vi "Data_Acquisition(I&O).vi"() -> ()   [LabVIEW 2020]
uses:
  <vilib>/Platform/TimedLoop/XDataNode/timing_clust.ctl
  <vilib>/Platform/TimedLoop/XDataNode/nitl_modes.ctl
  <vilib>/Platform/TimedLoop/XDataNode/wakeup.ctl
  <vilib>/FPGAPlugInAG/cRIO-9047/niLvFpga_Open_cRIO-9047.vi
  <vilib>/rvi/interface/common/dynamic/niFpgaDynamicAddResources.vi
  <vilib>/FPGAPlugInAG/Dynamic/niLvFpga_Download_Dynamic.vi
  <vilib>/FPGAPlugInAG/Dynamic/niLvFpga_Reset_Dynamic.vi
  <vilib>/FPGAPlugInAG/Dynamic/niLvFpga_Run_Dynamic.vi
  <vilib>/Utility/error.llb/Error Cluster From Error Code.vi
  <vilib>/rvi/errors/niLvFpgaAdjustHostInterfaceError.vi
  <vilib>/FPGAPlugInAG/Dynamic/niLvFpga_Close_Dynamic.vi
  <vilib>/Platform/TimedLoop/XDataNode/XDataNode.xnode
  <vilib>/rvi/interface/nirviOpenFPGA/nirviOpenFPGA.xnode
  FPGA_Link.vi
  <vilib>/rvi/interface/nirviMethod/nirviMethod.xnode
  <vilib>/rvi/interface/nirviReadWriteControl/nirviReadWriteControl.xnode
  <vilib>/rvi/interface/nirviCloseFPGA/nirviCloseFPGA.xnode
  <vilib>/Platform/TimedLoop/XDataNode/XDNodeRunTimeDep.lvlib
  <vilib>/rvi/interface/Simulation/niFpgaSimulationCallBeginRW.vi
  NiFpgaLv.dll
panel:
  out "Swing_Joint_Pi":fxp<+/-,24,5>
  out "Swing_Joint_Po":fxp<+/-,24,5>
  out "Boom_Joint_Pi":fxp<+/-,24,5>
  out "Boom_Joint_Po":fxp<+/-,24,5>
  out "Stick_Joint_Pi":fxp<+/-,48,10>
  out "Stick_Joint_Po":fxp<+/-,24,5>
  out "Reference_Pressure":fxp<+/-,24,5>
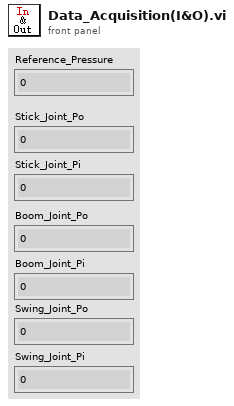
[diagram p1: front panel]
types:
  T1 = typedef "XDNodeRunTimeDep.lvlib/timing_clust.ctl" = cluster{"Expected End [f-1]":u64, "Actual End [f-1]":u64, "Finished Late? [f-1]":bool, "Expected End [i-1]":u64, "Actual End [i-1]":u64, "Finished Late? [i-1]":bool, "Expected Start [i]":u64, "Actual Start [i]":u64, "Expected Start [f]":u64, "Actual Start [f]":u64, "Source Name":string, "Structure Name":string, "Period":i64, "Deadline":i64, "Offset":i64, "Start":i64, "Priority":i32, "Timeout":i32, "Mode":T2, "Wakeup Reason":T3, "Error":errorcluster, "Source Type":string, "Secondary Source Type":string, "Global End Time":u64, "Global Start Time":u64, "Frame Duration":u64, "Iteration Duration":u64, "Assigned CPU":i32, "I/O Scan Engine Mode":u32}
  T2 = typedef "XDNodeRunTimeDep.lvlib/nitl_modes.ctl" = enum32{"No Change", "Process missed periods, maintain original phase", "Discard missed periods, maintain original phase", "Process missed periods, ignore original phase", "Discard missed periods, ignore original phase"}
  T3 = typedef "XDNodeRunTimeDep.lvlib/wakeup.ctl" = enum32{"Normal", "Aborted", "Asynchronous wakeup", "Timing source error", "Timed loop error", "Timeout"}
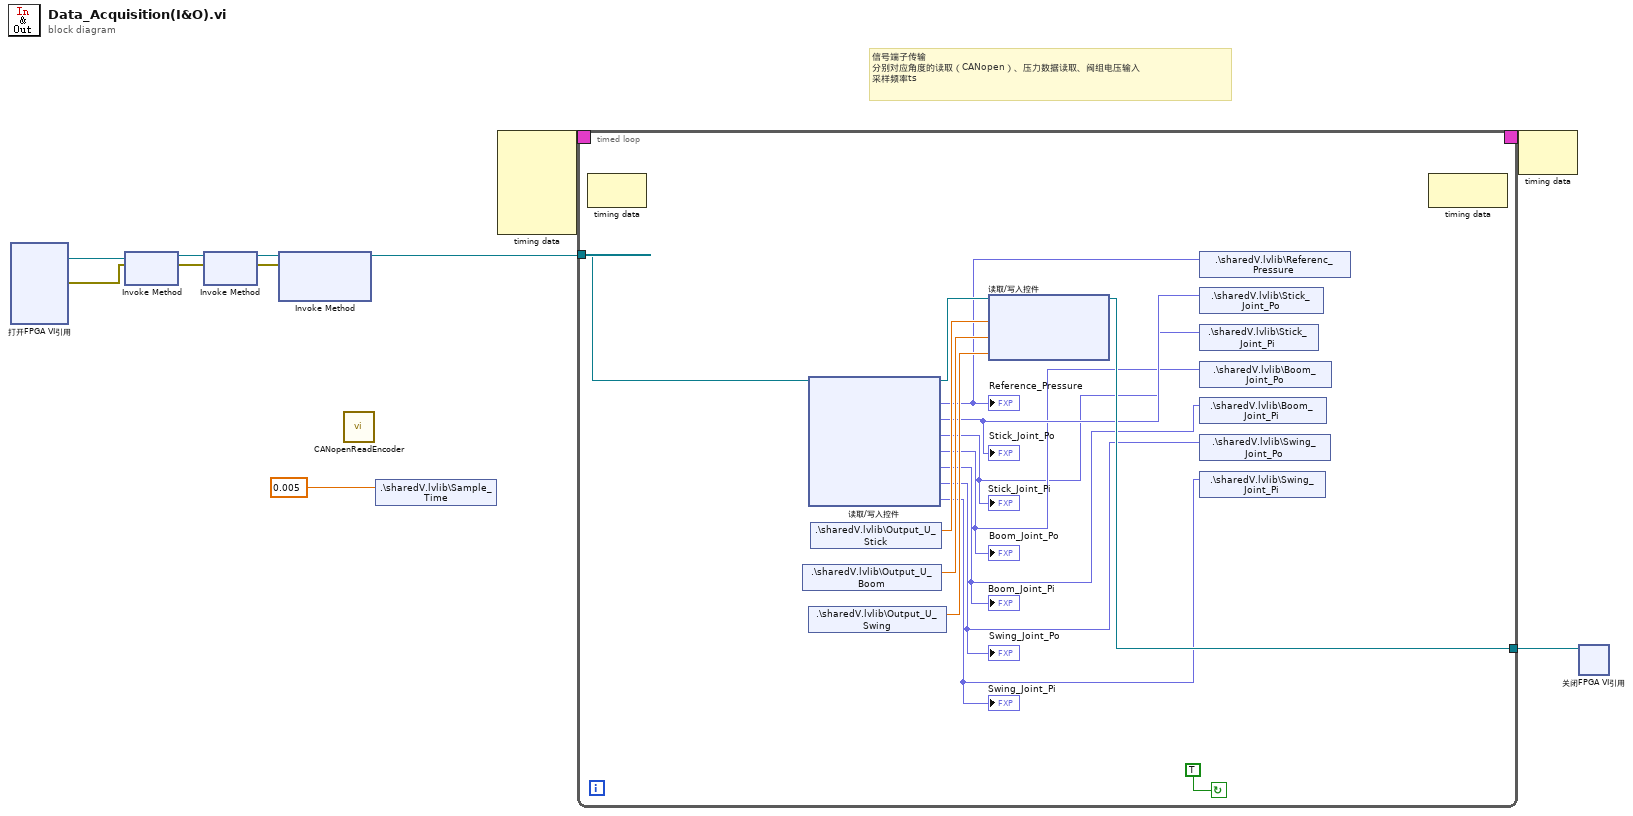
[diagram p0: block diagram]
diagram:
  # "信号端子传输\n分别对应角度的读取（CANopen）、压力数据读取、阀组电压输入\n采样频率ts"
  n1 = xnode "打开FPGA VI引用"() -> ("FPGA VI引用输出"=w9:refnum<k20>, "错误输出"=w6:errorcluster)  [unwired: 2 in]
  n2 = xnode "Invoke Method"("FPGA VI引用输入"=w9, "错误输入"=w6) -> ("FPGA VI引用输出"=w8:refnum<k20>, "错误输出"=w5:errorcluster)
  n3 = xnode "Invoke Method"("FPGA VI引用输入"=w8, "错误输入"=w5) -> ("FPGA VI引用输出"=w7:refnum<k20>, "错误输出"=w4:errorcluster)
  n4 = xnode "Invoke Method"("FPGA VI引用输入"=w7, "错误输入"=w4) -> ("FPGA VI引用输出"=w3:refnum<k20>)  [unwired: 1 in, 1 out]
  n5 = call "CANopenReadEncoder.vi"() -> ()  [unwired: 3 in]
  n6 = shared-variable ".\\sharedV.lvlib\\Sample_Time"(0.005) -> ()  [unwired: 1 in, 1 out]
  n7 = node-c288() -> (w11:T1)  [unwired: 5 in]
  n8 = timed-loop {
    timing: w11 -> [_]
    timing-out: [_] -> w10
    tunnel: w3 -> [w25]
    tunnel: [w23] -> w1
    stop <- TRUE continue-if-true
    n9 = node-c288() -> ()  [unwired: 1 in, 1 out]
    n10 = shared-variable ".\\sharedV.lvlib\\Output_U_Boom"() -> (w20:dbl)  [unwired: 1 in, 1 out]
    n11 = xnode "读取/写入控件"("FPGA VI引用输入"=w25) -> ("FPGA VI引用输出"=w24:refnum<k20>, "Reference_Pressure"=w18:fxp<+/-,24,5>, "Stick_Joint_Po"=w17:fxp<+/-,24,5>, "Stick_Joint_Pi"=w12:fxp<+/-,48,10>, "Boom_Joint_Po"=w13:fxp<+/-,24,5>, "Boom_Joint_Pi"=w14:fxp<+/-,24,5>, "Swing_Joint_Po"=w15:fxp<+/-,24,5>, "Swing_Joint_Pi"=w16:fxp<+/-,24,5>)  [unwired: 1 in, 1 out]
    "Reference_Pressure" <- w18
    "Stick_Joint_Po" <- w17
    "Stick_Joint_Pi" <- w12
    "Boom_Joint_Po" <- w13
    "Boom_Joint_Pi" <- w14
    "Swing_Joint_Po" <- w15
    "Swing_Joint_Pi" <- w16
    n12 = shared-variable ".\\sharedV.lvlib\\Output_U_Swing"() -> (w19:dbl)  [unwired: 1 in, 1 out]
    n13 = shared-variable ".\\sharedV.lvlib\\Output_U_Stick"() -> (w21:dbl)  [unwired: 1 in, 1 out]
    n14 = xnode "读取/写入控件"("FPGA VI引用输入"=w24, "Stick_Joint_Input"=w21, "Boom_Joint_Input"=w20, "Swing_Joint_Input"=w19) -> ("FPGA VI引用输出"=w23:refnum<k20>)  [unwired: 1 in, 1 out]
    n15 = shared-variable ".\\sharedV.lvlib\\Referenc_Pressure"(w18) -> ()  [unwired: 1 in, 1 out]
    n16 = shared-variable ".\\sharedV.lvlib\\Stick_Joint_Po"(w17) -> ()  [unwired: 1 in, 1 out]
    n17 = shared-variable ".\\sharedV.lvlib\\Stick_Joint_Pi"(w12) -> ()  [unwired: 1 in, 1 out]
    n18 = shared-variable ".\\sharedV.lvlib\\Boom_Joint_Po"(w13) -> ()  [unwired: 1 in, 1 out]
    n19 = shared-variable ".\\sharedV.lvlib\\Boom_Joint_Pi"(w14) -> ()  [unwired: 1 in, 1 out]
    n20 = shared-variable ".\\sharedV.lvlib\\Swing_Joint_Po"(w15) -> ()  [unwired: 1 in, 1 out]
    n21 = shared-variable ".\\sharedV.lvlib\\Swing_Joint_Pi"(w16) -> ()  [unwired: 1 in, 1 out]
    n22 = node-c288() -> ()  [unwired: 1 in, 1 out]
  }
  n23 = node-c288(w10) -> ()  [unwired: 1 out]
  n24 = xnode "关闭FPGA VI引用"("FPGA VI引用输入"=w1) -> ()  [unwired: 1 in, 1 out]
